vi "Read.vi"(11 "stream control":refnum<class "niUSRP Stream Control (DMA) v1 FPGA.lvclass">, 12 "ready for output":bool) -> (4 "data out":T1[](array[typedef]), 10 "output valid":bool, 15 "stream control":refnum<class "niUSRP Stream Control (DMA) v1 FPGA.lvclass">)   [LabVIEW 2025, in "niUSRP Stream Control (DMA) v1 FPGA.lvclass"]
uses:
  niUSRP Stream Control (DMA) v1 FPGA.lvclass
  <instrlib>/_niInstr/DSP/v1/Shared/Public/IQ Data.ctl
  niUSRP Stream Control (DMA) v1 FPGA.lvclass/niUSRP Stream Control (DMA) v1 FPGA.ctl
  <vilib>/rvi/DataTransferAndStorage/Container/Common/niFpgaContainerExecOnDevCompGetState.vi
  <vilib>/rvi/Emulation/niFpgaEmulationIsFPGAContextNoSignature.vi
  <vilib>/rvi/DataTransferAndStorage/Container/Common/niFpgaContainerGetUniqueNameForEmu.vi
  <vilib>/rvi/Memory/Memory_Emulation/niFpgaMemoryEmulationCacheClearOnFirstRun.vi
  <vilib>/rvi/Memory/Memory_Emulation/nirvimemoryEmulationManagerCache_MakeExclusive.vi
  <vilib>/rvi/Memory/Memory_Emulation/niFpgaMemoryEmulationValidateCache.vi
  <vilib>/rvi/Memory/Memory_Emulation/nirvimemoryEmulationManagerCache_InsertValue.vi
  <vilib>/Utility/error.llb/Clear Errors.vi
  <vilib>/rvi/Memory/Memory_Emulation/nirvimemoryEmulationManagerCache_ReleaseExclusive.vi
  <vilib>/rvi/Memory/Memory_Emulation/nirvimemoryEmulationManagerCache_GetValue.vi
  <vilib>/rvi/Memory/Memory_Emulation/nirvimemoryEmulationManagerCache_SetValue.vi
  <vilib>/rvi/Emulation/niFpgaProcessEmulError.vi
  <vilib>/rvi/Emulation/niFpgaSctlEmulationGetInTimedLoop.vi
  <instrlib>/_niInstr/DSP/v1/FPGA/Public/Sub VIs/Data Conversion/U32 to IQ - N spc - S18.1.vi
  <vilib>/rvi/DataTransferAndStorage/Container/XNode/niFpgaContainer.xnode
  <vilib>/rvi/DataTransferAndStorage/Register/Emulation/niFpgaRegisterEmulationRefIn.vi
  <instrlib>/_niInstr/Basic Elements/v1/FPGA/niInstr Basic Elements v1 FPGA.lvlib
  <instrlib>/_niInstr/DSP/v1/FPGA/niInstr DSP v1 FPGA.lvlib
  <instrlib>/_niInstr/DSP/v1/Shared/niInstr DSP v1 Shared.lvlib
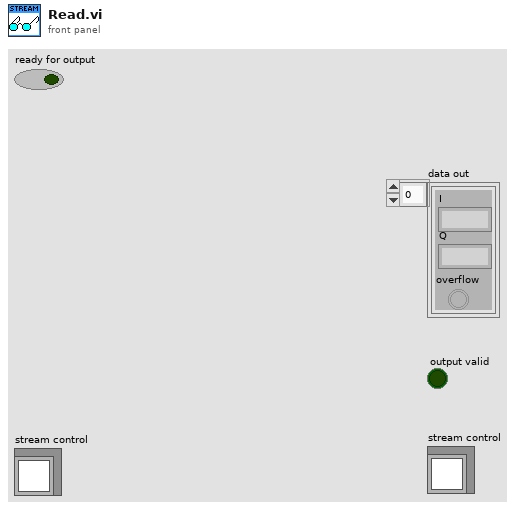
[diagram p1: front panel]
types:
  T1 = typedef "niInstr DSP v1 Shared.lvlib/IQ Data.ctl" = cluster{"I":fxp<+/-,18,1>, "Q":fxp<+/-,18,1>, "overflow":bool}
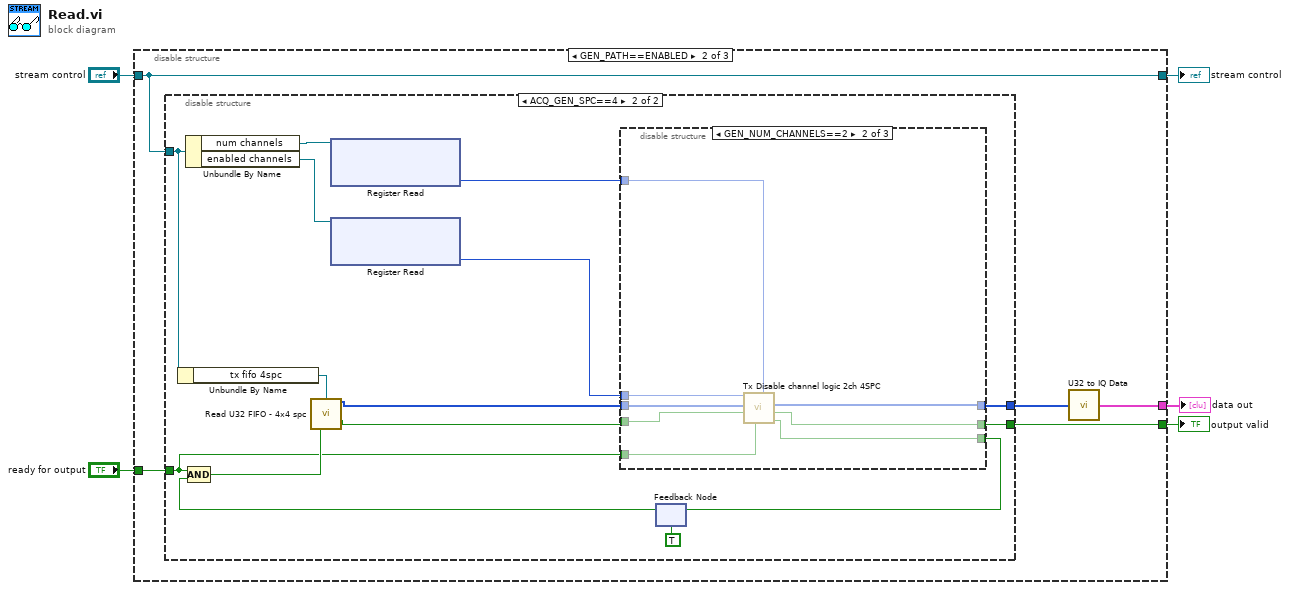
[diagram p0: block diagram]
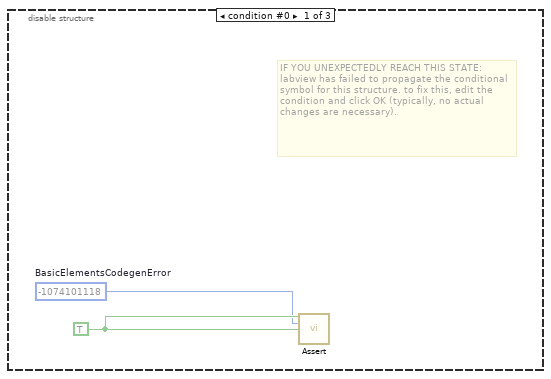
[diagram p2: hidden frame]
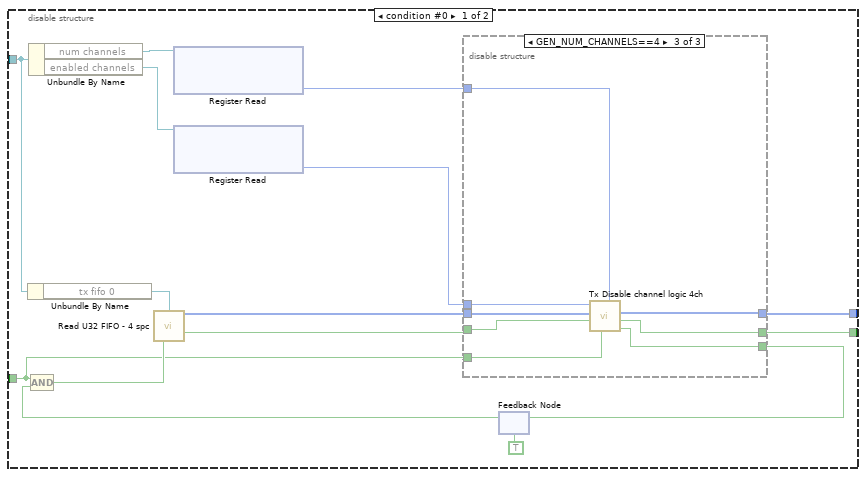
[diagram p3: hidden frame]
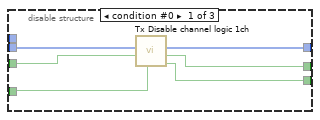
[diagram p4: hidden frame]
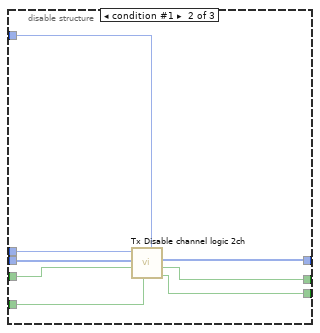
[diagram p5: hidden frame]
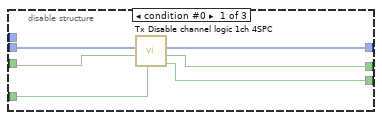
[diagram p6: hidden frame]
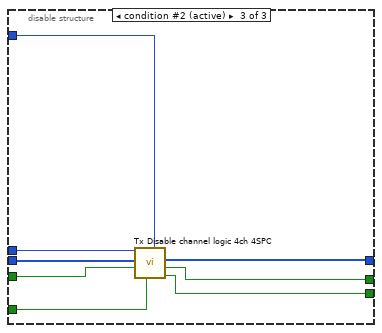
[diagram p7: hidden frame]
diagram:
  n1 = disable-structure shown="GEN_PATH==ENABLED" {
    disable-tunnel: "stream control" -> [_ w11 _]
    disable-tunnel: [_ w11 _] -> w4
    disable-tunnel: [_ w12 _] -> w3
    disable-tunnel: "ready for output" -> [_ w10 _]
    disable-tunnel: [_ w8 _] -> w1
    frame condition #0 {
      w7 = TRUE ("assert")
      w6 = -1074101118  # BasicElementsCodegenError
      # "IF YOU UNEXPECTEDLY REACH THIS STATE:\nlabview has failed to propagate the conditional symbol for this structure. to fix this, edit the condition and click OK (typically, no actual changes are necessary)."
      n2 = call <instrlib>:"Assert.vi"("assert"=w7, "error code"=w6, "enable show error"=w7) -> ()  [unwired: 13 in]
    }
    frame condition #1 (active) {
      n3 = disable-structure shown="ACQ_GEN_SPC==4" {
        disable-tunnel: [w26 w64] -> w12
        disable-tunnel: w11 -> [w21 w55]
        disable-tunnel: w10 -> [w13 w51]
        disable-tunnel: [w16 w56] -> w9
        frame condition #0 {
          n4 = Unbundle By Name(w21) -> ("tx fifo 0"=w15:refnum<k21>)
          n5 = Unbundle By Name(w21) -> ("num channels"=w20:refnum<k21>, "enabled channels"=w19:refnum<k21>)
          n6 = xnode ("Register Read")("Register In"=w20) -> ("Data"=w18:u32)  [unwired: 1 out]
          n7 = xnode ("Register Read")("Register In"=w19) -> ("Data"=w17:u32)  [unwired: 1 out]
          n8 = feedback #1(TRUE) -> (w22:bool)
          n9 = Compound Arithmetic op=AND(w13, w22) -> (w25:bool)
          n10 = call "Read U32 FIFO - 4 spc.vi"("fifo"=w15, "ready for output"=w25) -> ("output data"=w14:u32[], "output valid"=w27:bool)  [unwired: 12 in]
          n11 = disable-structure shown="GEN_NUM_CHANNELS==4" {
            disable-tunnel: [w31 w38 w45] -> w26
            disable-tunnel: [w32 w39 w46] -> w16
            disable-tunnel: w27 -> [w29 w35 w43]
            disable-tunnel: [w30 w37 w44] -> w23
            disable-tunnel: w18 -> [_ w41 w49]
            disable-tunnel: w17 -> [_ w36 w48]
            disable-tunnel: w14 -> [w33 w40 w47]
            disable-tunnel: w13 -> [w28 w34 w42]
            frame condition #0 {
              n12 = call "Tx Disable channel logic 1ch.vi"("ready for output"=w28, "input valid"=w29, "data in"=w33) -> ("enable new data"=w30:bool, "output valid"=w31:bool, "data out"=w32:u32[])  [unwired: 6 in]
            }
            frame condition #1 {
              n13 = call "Tx Disable channel logic 2ch.vi"("num channels"=w41, "ready for output"=w34, "input valid"=w35, "data in"=w40, "enabled channels"=w36) -> ("enable new data"=w37:bool, "output valid"=w38:bool, "data out"=w39:u32[])  [unwired: 4 in]
            }
            frame condition #2 (active) {
              n14 = call "Tx Disable channel logic 4ch.vi"("num channels"=w49, "ready for output"=w42, "input valid"=w43, "data in"=w47, "enabled channels"=w48) -> ("enable new data"=w44:bool, "output valid"=w45:bool, "data out"=w46:u32[])  [unwired: 4 in]
            }
          }
          n15 = feedback-in #1(w23) -> ()
        }
        frame condition #1 (active) {
          n16 = Unbundle By Name(w55) -> ("tx fifo 4spc"=w54:refnum<k21>)
          n17 = Unbundle By Name(w55) -> ("num channels"=w60:refnum<k21>, "enabled channels"=w59:refnum<k21>)
          n18 = xnode ("Register Read")("Register In"=w60) -> ("Data"=w58:u32)  [unwired: 1 out]
          n19 = xnode ("Register Read")("Register In"=w59) -> ("Data"=w57:u32)  [unwired: 1 out]
          n20 = feedback #2(TRUE) -> (w61:bool)
          n21 = Compound Arithmetic op=AND(w51, w61) -> (w53:bool)
          n22 = call "Read U32 FIFO - 4x4 spc.vi"("fifo"=w54, "ready for output"=w53) -> ("output data"=w50:u32[], "output valid"=w52:bool)  [unwired: 12 in]
          n23 = disable-structure shown="GEN_NUM_CHANNELS==2" {
            disable-tunnel: [w69 w77 w82] -> w64
            disable-tunnel: [w67 w71 w83] -> w56
            disable-tunnel: w52 -> [w66 w73 w80]
            disable-tunnel: [w68 w76 w81] -> w62
            disable-tunnel: w58 -> [_ w75 w86]
            disable-tunnel: w57 -> [_ w74 w85]
            disable-tunnel: w50 -> [w70 w78 w84]
            disable-tunnel: w51 -> [w65 w72 w79]
            frame condition #0 {
              n24 = call "Tx Disable channel logic 1ch 4SPC.vi"("ready for output"=w65, "input valid"=w66, "data in"=w70) -> ("enable new data"=w68:bool, "output valid"=w69:bool, "data out"=w67:u32[])  [unwired: 6 in]
            }
            frame condition #1 {
              n25 = call "Tx Disable channel logic 2ch 4SPC.vi"("num channels"=w75, "ready for output"=w72, "input valid"=w73, "data in"=w78, "enabled channels"=w74) -> ("enable new data"=w76:bool, "output valid"=w77:bool, "data out"=w71:u32[])  [unwired: 4 in]
            }
            frame condition #2 (active) {
              n26 = call "Tx Disable channel logic 4ch 4SPC.vi"("num channels"=w86, "ready for output"=w79, "input valid"=w80, "data in"=w84, "enabled channels"=w85) -> ("enable new data"=w81:bool, "output valid"=w82:bool, "data out"=w83:u32[])  [unwired: 4 in]
            }
          }
          n27 = feedback-in #2(w62) -> ()
        }
      }
      n28 = call-poly <instrlib>:"U32 to IQ Data.vi"("U32 data"=w9) -> ("IQ data"=w8:T1[])  [unwired: 14 in]
    }
    frame condition #2 {
    }
  }
  "stream control" <- w4
  "output valid" <- w3
  "data out" <- w1
